vi "Get Arm Pot.vi"() -> (3 "Normalized Value":dbl)   [LabVIEW 2015]
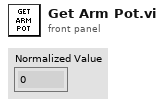
[diagram p1: front panel]
types:
  T1 = typedef "WPI_PotentiometerDevRef.ctl" = cluster{"DevStatus":errorcluster, "Analog Channel":T2, "Invert Output":bool}
  T2 = typedef "FPGA_AIChannel.ctl" = enum8{"AI 0", "AI 1", "AI 2", "AI 3", "AI MXP 0", "AI MXP 1", "AI MXP 2", "AI MXP 3", "Invalid"}
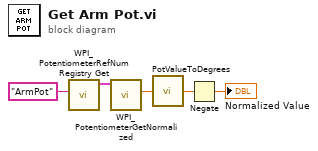
[diagram p0: block diagram]
diagram:
  n1 = call <vilib>:"WPI_PotentiometerRefNum Registry Get.vi"("refnum name"="ArmPot") -> ("PotDevRef"=w5:T1)  [unwired: 9 in, 1 out]
  n2 = call <vilib>:"WPI_PotentiometerGetNormalized.vi"("PotDevRef"=w5) -> ("Normalized Value"=w1:dbl)  [unwired: 8 in, 2 out]
  n3 = call "PotValueToDegrees.vi"("PotIn"=w1) -> ("Degrees"=w3:dbl)  [unwired: 1 in]
  n4 = Negate(x=w3) -> (-x=→"Normalized Value":dbl)
